vi "Horizon Line Color Write 9.vi"(4 "error in (no error)":errorcluster, 5 "Value":u32(colorbox)=16777225, 6 "Container State":T4, 7 "Display State In":T1={"Draw Options"={"Text Color"=16777238, "Wing Color"=16751616, "Dial Outline Color"=13816530, "Sky Color"=3381759, "Ground Color"=8213043, "Horizon Line Color"=16777225, "Outline Color"=0, "Dial Background Color"=5987163, "Draw Wings"=TRUE, "Draw Text"=TRUE, "Font Name"="Helvetica", "Angle units"=enum."Degrees"}}) -> (0 "error out":errorcluster, 3 "Display State Out":T1={"Draw Options"={"Text Color"=16777238, "Wing Color"=16751616, "Dial Outline Color"=13816530, "Sky Color"=3381759, "Ground Color"=8213043, "Horizon Line Color"=16777225, "Outline Color"=0, "Dial Background Color"=5987163, "Draw Wings"=TRUE, "Draw Text"=TRUE, "Font Name"="Helvetica", "Angle units"=enum."Degrees"}})   [LabVIEW 2017, in "Attitude Indicator.xctl"]
uses:
  <vilib>/robotics/Controls/Attitude Indicator/Attitude Indicator.xctl
  <vilib>/_xctls/Container State.ctl
  <vilib>/robotics/Controls/Attitude Indicator/_Attitude Indicator Support Files/Attitude Indicator State.ctl
  <vilib>/robotics/Controls/Attitude Indicator/Attitude Picture/Draw Options.ctl
  <vilib>/robotics/Controls/Utilities/Angle Units.ctl
  <vilib>/_xctls/XControlSupport.lvlib
  <vilib>/robotics/Controls/Attitude Indicator/Attitude Picture/NI_Robotics_Attitude Picture.lvlib
  <vilib>/robotics/Controls/Utilities/NI_Robotics_Control Utilities.lvlib
panel:
  # "Replace the Value Control below with a Control of desired type.\nDo not remove this Control or the others from the connector pane.\nDo not change the connector pane pattern.\nThe Value control should always be the third terminal from top on the input side in the connector pane."
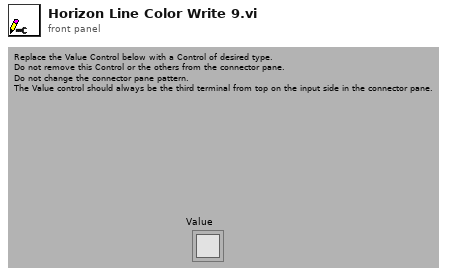
[diagram p1: front panel]
types:
  T1 = typedef "Attitude Indicator.xctl/Attitude Indicator State.ctl" = cluster{"Draw Options":T2}
  T2 = typedef "NI_Robotics_Attitude Picture.lvlib/Draw Options.ctl" = cluster{"Text Color":u32, "Wing Color":u32, "Dial Outline Color":u32, "Sky Color":u32, "Ground Color":u32, "Horizon Line Color":u32, "Outline Color":u32, "Dial Background Color":u32, "Draw Wings":bool, "Draw Text":bool, "Font Name":string, "Angle units":T3}
  T3 = typedef "NI_Robotics_Control Utilities.lvlib/Angle Units.ctl" = enum16{"Radians", "Degrees"}
  T4 = typedef "XControlSupport.lvlib/Container State.ctl" = cluster{"Indicator?":bool, "Run Mode?":bool, " Refnum":refnum<vi>}
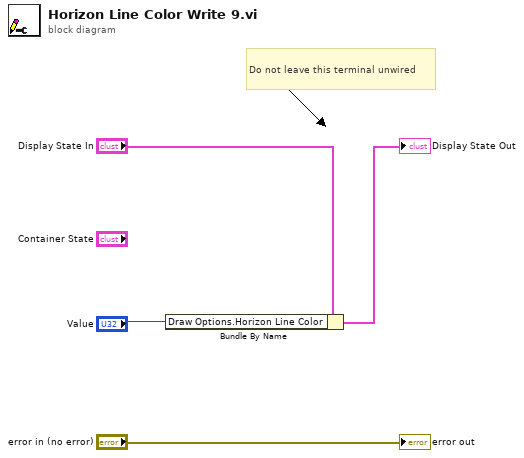
[diagram p0: block diagram]
diagram:
  # "Do not leave this terminal unwired"
  n1 = Bundle By Name(cluster="Display State In", "Draw Options.Horizon Line Color"="Value") -> (→"Display State Out":T1)
  "error out" <- "error in (no error)"
